vi "CreateDevice_8532.vi"(8 "error in (no error)":errorcluster) -> (0 "error out":errorcluster, 3 "hDevice":i32)   [LabVIEW 2009]
uses:
  PCI8532_32.dll
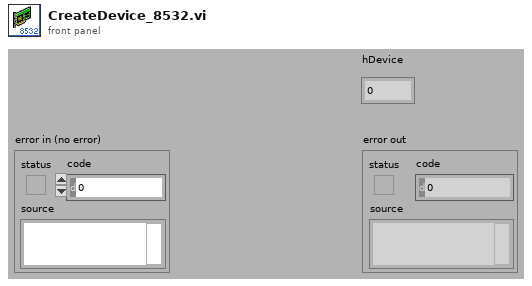
[diagram p1: front panel]
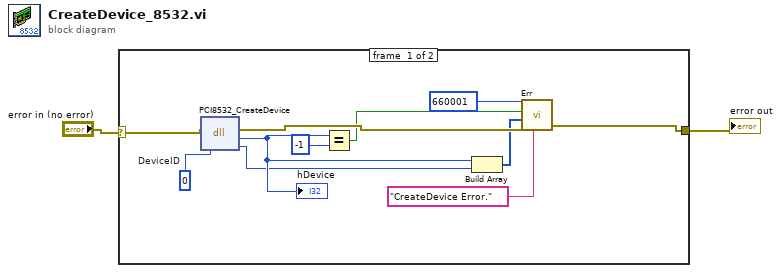
[diagram p0: block diagram]
diagram:
  n1 = case shown="无错误" "error in (no error)" {
    selector: "error in (no error)" -> [w11 w14]
    tunnel: [w8 w14] -> w1
    frame #0 {
      w12 = 0  # DeviceID
      n2 = dll-call lib="PCI8532_32.dll" fn="PCI8532_CreateDevice" label="CreateDevice"(error in=w11, "DeviceID"=w12) -> (error out=w10:errorcluster, "返回类型"=w7:i32, "DeviceID"=w6:i32)  [unwired: 2 in, 1 out]
      "hDevice" <- w7
      n3 = Equal?(x=w7, y=-1) -> (x = y?=w9:bool)
      n4 = Build Array(w7, w6) -> (w5:i32[])
      n5 = call "Err.vi"("source"="CreateDevice Error.", "error in (no error)"=w10, "Par"=w5, "error?"=w9, "code"=660001) -> ("error out"=w8:errorcluster)  [unwired: 6 out]
    }
    frame #1 {
    }
  }
  "error out" <- w1
